vi "Create mailbox.vi"(4 "error in (no error)":errorcluster, 5 "max queue size (-1, unlimited)":i32, 7 "name (unnamed)":string) -> (0 "error out":errorcluster, 1 "created new?":bool, 3 "Mailbox ref":T1)   [LabVIEW 2021, in "Queued messenger.lvlib"]
doc: "Wrapped [Obtain queue.vi] to create a mailbox."
uses:
  <userlib>/Queued messenger lib/Queued messenger.lvlib
  <userlib>/Queued messenger lib/TypeDefs/Mailbox ref.ctl
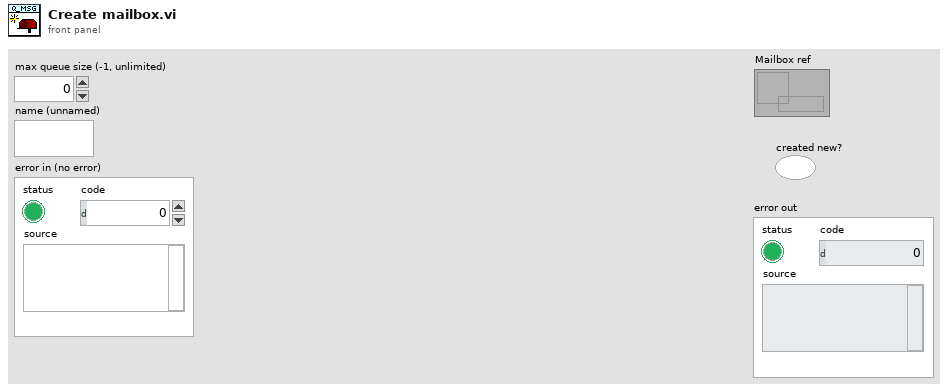
[diagram p1: front panel]
types:
  T1 = typedef "Queued messenger.lvlib/Mailbox ref.ctl" = refnum<queue>
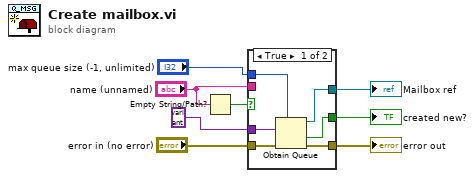
[diagram p0: block diagram]
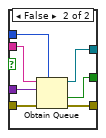
[diagram p2: hidden frame]
diagram:
  n1 = Empty String/Path?(string/path="name (unnamed)") -> (empty?=w3:bool)
  n2 = case shown="True" w3 {
    tunnel: variant -> [w9 w21]
    tunnel: "max queue size (-1, unlimited)" -> [w14 w20]
    tunnel: "name (unnamed)" -> [_ w19]
    tunnel: "error in (no error)" -> [w13 w18]
    tunnel: [w12 w17] -> w5
    tunnel: [w11 w16] -> w4
    tunnel: [w10 w15] -> w1
    frame True {
      n3 = Obtain Queue(max queue size (-1, unlimited)=w14, element data type=w9, error in (no error)=w13) -> (queue out=w10:refnum<queue>, created new?=w11:bool, error out=w12:errorcluster)  [unwired: 2 in]
    }
    frame False {
      n4 = Obtain Queue(max queue size (-1, unlimited)=w20, name (unnamed)=w19, element data type=w21, error in (no error)=w18) -> (queue out=w15:refnum<queue>, created new?=w16:bool, error out=w17:errorcluster)  [unwired: 1 in]
    }
  }
  "error out" <- w5
  "created new?" <- w4
  "Mailbox ref" <- w1
